vi "MKS670_GPIB_init.vi"(8 "error in (no error)":errorcluster, 11 "GPIB Address":string) -> (0 "error out":errorcluster, 2 "Device Version":dbl, 3 "GPIB out":string, 4 "status":bool, 5 "Device Name":string)   [LabVIEW 2019]
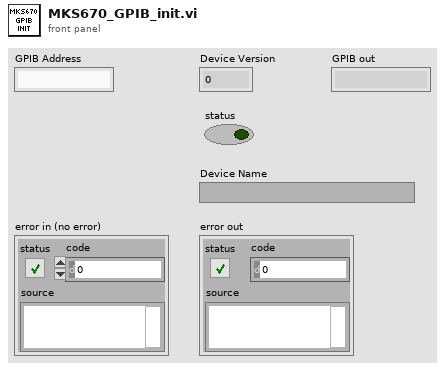
[diagram p1: front panel]
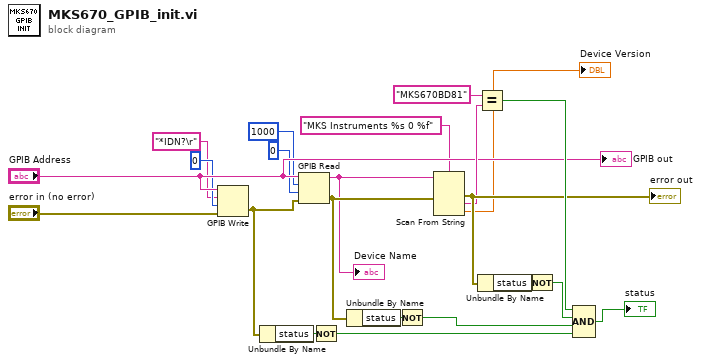
[diagram p0: block diagram]
diagram:
  n1 = GPIB Write(0:"GPIB Address", 1:"*IDN?\r" ("data"), 2:0, 3:"error in (no error)") -> (6:w12:errorcluster)  [unwired: 1 in, 1 out]
  n2 = Unbundle By Name(w12) -> ("status"=w14:bool)
  n3 = GPIB Read(0:"GPIB Address", 1:1000 ("byte count"), 2:0, 3:w12) -> (5:w3:string, 7:w13:errorcluster)  [unwired: 1 in, 1 out]
  "Device Name" <- w3
  n4 = Not(x=w14) -> (.not. x?=w18:bool)
  n5 = Unbundle By Name(w13) -> ("status"=w16:bool)
  n6 = Not(x=w16) -> (.not. x?=w19:bool)
  n7 = Scan From String(format string="MKS Instruments %s 0 %f", input string=w3, error in=w13) -> (error out=w15:errorcluster, output 1=w11:string, output 2=→"Device Version":dbl)  [unwired: 3 in, 2 out]
  "error out" <- w15
  n8 = Equal?(x="MKS670BD81" ("y"), y=w11) -> (x = y?=w20:bool)
  n9 = Unbundle By Name(w15) -> ("status"=w17:bool)
  n10 = Not(x=w17) -> (.not. x?=w21:bool)
  n11 = Compound Arithmetic op=AND(w20, w21, w19, w18) -> (→"status":bool)
  "GPIB out" <- "GPIB Address"
